vi "String2XNETsignal.vi"(0 "X-netString":string) -> (14 "DBC_XnetSignal":refnum<k21>)   [LabVIEW 2020, in "Abstract_Diagnose.lvclass"]
uses:
  Abstract_Diagnose_class/Abstract_Diagnose.lvclass
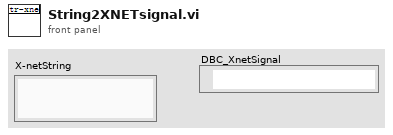
[diagram p1: front panel]
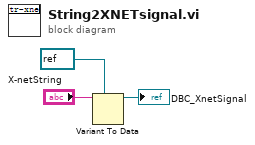
[diagram p0: block diagram]
diagram:
  n1 = Variant To Data(type=refnum<k21> refnum ("类型"), Variant="X-netString") -> (data=→"DBC_XnetSignal":refnum<k21>)  [unwired: 1 in, 1 out]
